vi "Associated Power Technologies 8500 Series List Mode.vi"() -> ()   [LabVIEW 2014]
doc: "This VI is an example for controlling the power source, APT-8500 series, of Associated Power Technologies. \n\nThe list mode which behave the configured sequences step by step is one of the operation mode on APT8500. This VI is an example showing how many configurations need to be set up."
uses:
  <instrlib>/Associated Power Technologies 8500 Series/Public/Configure/List Mode/List Mode - Delete File.vi
  <instrlib>/Associated Power Technologies 8500 Series/Public/Configure/List Mode/List Mode - Add File.vi
  <instrlib>/Associated Power Technologies 8500 Series/Public/Configure/List Mode/List Mode - Edit File.vi
  <instrlib>/Associated Power Technologies 8500 Series/Public/Configure/List Mode/List Mode - Configure File Loop.vi
  <instrlib>/Associated Power Technologies 8500 Series/Public/Configure/List Mode/List Mode - Configure Trigger Source.vi
  <instrlib>/Associated Power Technologies 8500 Series/Public/Configure/List Mode/List Mode - Configure Base.vi
  <instrlib>/Associated Power Technologies 8500 Series/Public/Configure/List Mode/List Mode - Configure Range.vi
  <instrlib>/Associated Power Technologies 8500 Series/Public/Configure/List Mode/List Mode - Configure General AC Voltage.vi
  <instrlib>/Associated Power Technologies 8500 Series/Public/Configure/List Mode/List Mode - Configure General Frequency.vi
  <instrlib>/Associated Power Technologies 8500 Series/Public/Configure/List Mode/List Mode - Configure General DC Voltage.vi
  <instrlib>/Associated Power Technologies 8500 Series/Public/Configure/List Mode/List Mode - Configure Phase Connection.vi
  <instrlib>/Associated Power Technologies 8500 Series/Public/Configure/List Mode/List Mode - Seq - Add Sequence.vi
  <instrlib>/Associated Power Technologies 8500 Series/Public/Configure/List Mode/List Mode - Seq - Edit Sequence.vi
  <instrlib>/Associated Power Technologies 8500 Series/Public/Configure/List Mode/List Mode - Seq - Configure Output Waveform.vi
  <instrlib>/Associated Power Technologies 8500 Series/Public/Configure/List Mode/List Mode - Seq - Configure Start Angle.vi
  <instrlib>/Associated Power Technologies 8500 Series/Public/Configure/List Mode/List Mode - Seq - Configure Start AC Voltage.vi
  <instrlib>/Associated Power Technologies 8500 Series/Public/Configure/List Mode/List Mode - Seq - Configure Start Frequency.vi
  <instrlib>/Associated Power Technologies 8500 Series/Public/Configure/List Mode/List Mode - Seq - Configure Start DC Voltage.vi
  <instrlib>/Associated Power Technologies 8500 Series/Public/Configure/List Mode/List Mode - Seq - Configure End AC Voltage.vi
  <instrlib>/Associated Power Technologies 8500 Series/Public/Configure/List Mode/List Mode - Seq - Configure End Frequency.vi
  <instrlib>/Associated Power Technologies 8500 Series/Public/Configure/List Mode/List Mode - Seq - Configure End DC Voltage.vi
  <instrlib>/Associated Power Technologies 8500 Series/Public/Configure/List Mode/List Mode - Seq - Configure Cycle.vi
  <instrlib>/Associated Power Technologies 8500 Series/Public/Configure/List Mode/List Mode - Seq - Configure Dwell Time.vi
  <instrlib>/Associated Power Technologies 8500 Series/Public/Configure/List Mode/List Mode - Seq - Configure Time Unit.vi
  <instrlib>/Associated Power Technologies 8500 Series/Public/Configure/List Mode/List Mode - Seq - Configure Limitation Delay Time.vi
  <instrlib>/Associated Power Technologies 8500 Series/Public/Configure/List Mode/List Mode - Seq - Configure THD.vi
  <instrlib>/Associated Power Technologies 8500 Series/Public/Configure/List Mode/List Mode - Seq - Configure Current High Limitation.vi
  <instrlib>/Associated Power Technologies 8500 Series/Public/Configure/List Mode/List Mode - Seq - Configure Current Low Limitation.vi
  <instrlib>/Associated Power Technologies 8500 Series/Public/Configure/List Mode/List Mode - Seq - Configure Power High Limitation.vi
  <instrlib>/Associated Power Technologies 8500 Series/Public/Configure/List Mode/List Mode - Seq - Configure Power Low Limitation.vi
  <instrlib>/Associated Power Technologies 8500 Series/Public/Configure/List Mode/List Mode - Seq - Configure PF High Limitation.vi
  <instrlib>/Associated Power Technologies 8500 Series/Public/Configure/List Mode/List Mode - Seq - Configure PF Low Limitation.vi
  <instrlib>/Associated Power Technologies 8500 Series/Public/Configure/List Mode/List Mode - Seq - Configure Current Peak High Limitation.vi
  <instrlib>/Associated Power Technologies 8500 Series/Public/Configure/List Mode/List Mode - Seq - Configure Current Peak Low Limitation.vi
  <instrlib>/Associated Power Technologies 8500 Series/Public/Configure/List Mode/List Mode - Seq - Configure Reactive Power High Limitation.vi
  <instrlib>/Associated Power Technologies 8500 Series/Public/Configure/List Mode/List Mode - Seq - Configure Reactive Power Low Limitation.vi
  <instrlib>/Associated Power Technologies 8500 Series/Public/Configure/List Mode/List Mode - Seq - Configure Crest Factor High Limitation.vi
  <instrlib>/Associated Power Technologies 8500 Series/Public/Configure/List Mode/List Mode - Seq - Configure Crest Factor Low Limitation.vi
  <instrlib>/Associated Power Technologies 8500 Series/Public/Configure/List Mode/List Mode - Seq - Configure Apparent Power High Limitation.vi
  <instrlib>/Associated Power Technologies 8500 Series/Public/Configure/List Mode/List Mode - Seq - Configure Apparent Power Low Limitation.vi
  <instrlib>/Associated Power Technologies 8500 Series/Associated Power Technologies 8500 Series.lvlib
panel:
  in  "Sequences Array":T1(array[cluster])=[{"Waveform Type"=0, "Start Angle(degree)"=90, "Start AC Voltage"=100.0, "Start Frequency"=50.0, "Start DC Voltage"=0.0, "End AC Voltage"=120.0, "End Frequency"=60.0, "End DC Voltage"=0.0, "Cycles"=9999, "Dwell Time"=1.0, "Unit"=1, "Delay Time"=1.0, "THD"=0.0, "Limits"={"A-HI"=0.0, "A-LO"=0.0, "P-HI"=0, "P-LO"=0, "PF-HI"=0.0, "PF-LO"=0.0, "Apk-HI"=0.0, "Apk-LO"=0.0, "Q-HI"=0, "Q-LO"=0, "CF-HI"=0.0, "CF-LO"=0.0, "VA-HI"=0.0, "VA-LO"=0.0}}] {"Waveform Type" items=["Sine", "Triangle", "Square", "Clipped"]; "Start Angle(degree)" max=359; "Start AC Voltage" min=0.0 max=310.0; "Start Frequency" min=5.0 max=1200.0; "Start DC Voltage" min=0.0 max=420.0; "End AC Voltage" min=0.0 max=310.0; "End Frequency" min=5.0 max=1200.0; "End DC Voltage" min=0.0 max=420.0; "Cycles" min=1 max=9999; "Dwell Time" min=1.0 max=999.9 step=0.1; "Unit" items=["MS", "SECOND", "MINUTE", "HOUR"]; "Delay Time" min=0.0 max=999.9 step=0.1; "THD" min=0.0 max=46.0 step=0.1}
  in  "Program Setup":T2={"Loop Count"=1, "Trigger Source"=0, "Base"=1, "Range"=0, "AC Voltage"=100.0, "Frequency"=60.0, "DC Voltage"=0.0, "Phase Connection"=0} {"Loop Count" max=50000; "Trigger Source" items=["AUTO", "MANUAL"]; "Base" items=["TIME", "CYCLE"]; "Range" items=["AUTO", "HIGH", "LOW"]; "AC Voltage" min=0.0 max=310.0; "Frequency" min=5.0 max=1200.0; "DC Voltage" min=0.0 max=420.0; "Phase Connection" items=["OFF", "ON"]}
  in  "File Name":string="EXAMPLE"
  in  "Serial Configuration":T3={"Baud Rate"=115200, "Parity"=0, "Data Bits"=8, "Stop Bits"=10, "Flow Control"=0} {"Flow Control" items=["None", "XON/XOFF", "RTS/CTS", "XON/XOFF & RTS/CTS", "DTR/DSR", "XON/XOFF & DTR/DSR"]; "Stop Bits" items=["1.0"=10, "1.5"=15, "2.0"=20]; "Data Bits" items=["7"=7, "8"=8]; "Parity" items=["None", "Odd", "Even", "Mark", "Space"]; "Baud Rate" items=["300"=300, "600"=600, "1200"=1200, "2400"=2400, "4800"=4800, "9600"=9600, "19200"=19200, "38400"=38400, "115200"=115200]}
  in  "VISA resource name":refnum<visa-resource-name>
  # "Create List Mode File of APT-8500 Series"
  # "This program is to explain how to build up a List Mode file and configure the parameters."
  # "Initialization"
  # "Configurations"
  # "(c) 2020 Associated Power Technologies.  ALL RIGHTS RESERVED."
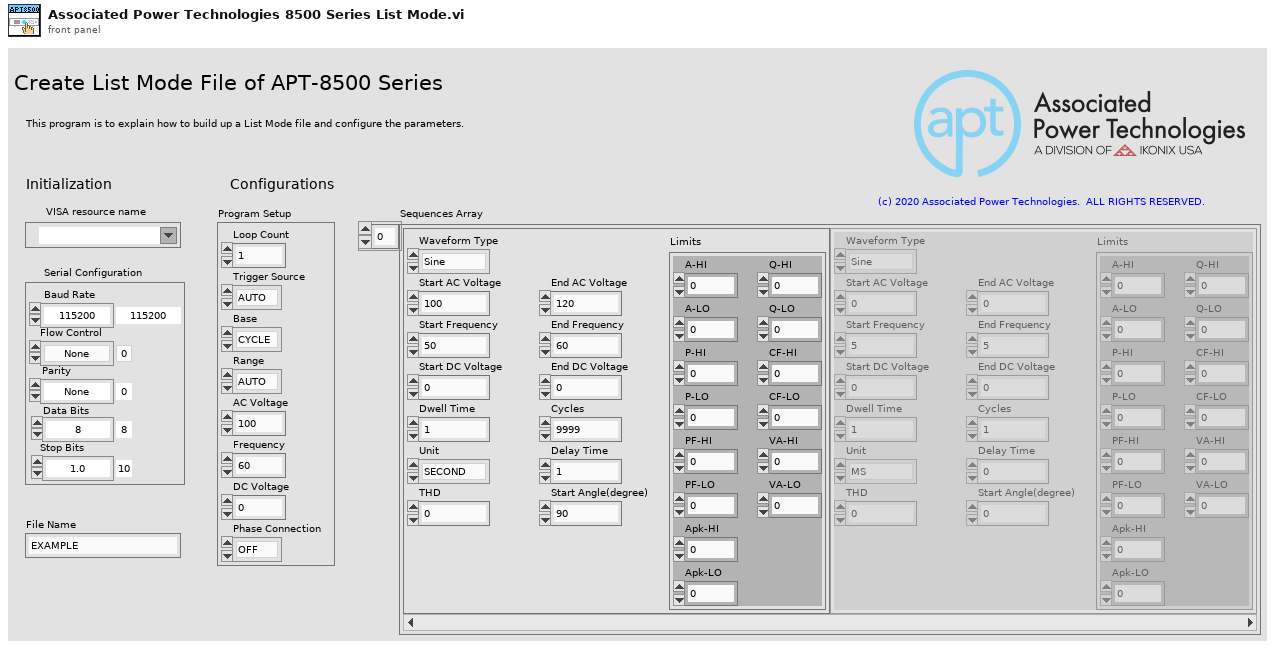
[diagram p1: front panel]
types:
  T1 = cluster{"Waveform Type":u16, "Start Angle(degree)":u16, "Start AC Voltage":dbl, "Start Frequency":dbl, "Start DC Voltage":dbl, "End AC Voltage":dbl, "End Frequency":dbl, "End DC Voltage":dbl, "Cycles":u32, "Dwell Time":dbl, "Unit":u16, "Delay Time":dbl, "THD":dbl, "Limits":cluster{"A-HI":dbl, "A-LO":dbl, "P-HI":u32, "P-LO":u32, "PF-HI":dbl, "PF-LO":dbl, "Apk-HI":dbl, "Apk-LO":dbl, "Q-HI":u32, "Q-LO":u32, "CF-HI":dbl, "CF-LO":dbl, "VA-HI":dbl, "VA-LO":dbl}}[]
  T2 = cluster{"Loop Count":u16, "Trigger Source":u16, "Base":u16, "Range":u16, "AC Voltage":dbl, "Frequency":dbl, "DC Voltage":dbl, "Phase Connection":u16}
  T3 = cluster{"Baud Rate":u32, "Parity":u16, "Data Bits":u16, "Stop Bits":u16, "Flow Control":u16}
  T4 = cluster{"A-HI":dbl, "A-LO":dbl, "P-HI":u32, "P-LO":u32, "PF-HI":dbl, "PF-LO":dbl, "Apk-HI":dbl, "Apk-LO":dbl, "Q-HI":u32, "Q-LO":u32, "CF-HI":dbl, "CF-LO":dbl, "VA-HI":dbl, "VA-LO":dbl}
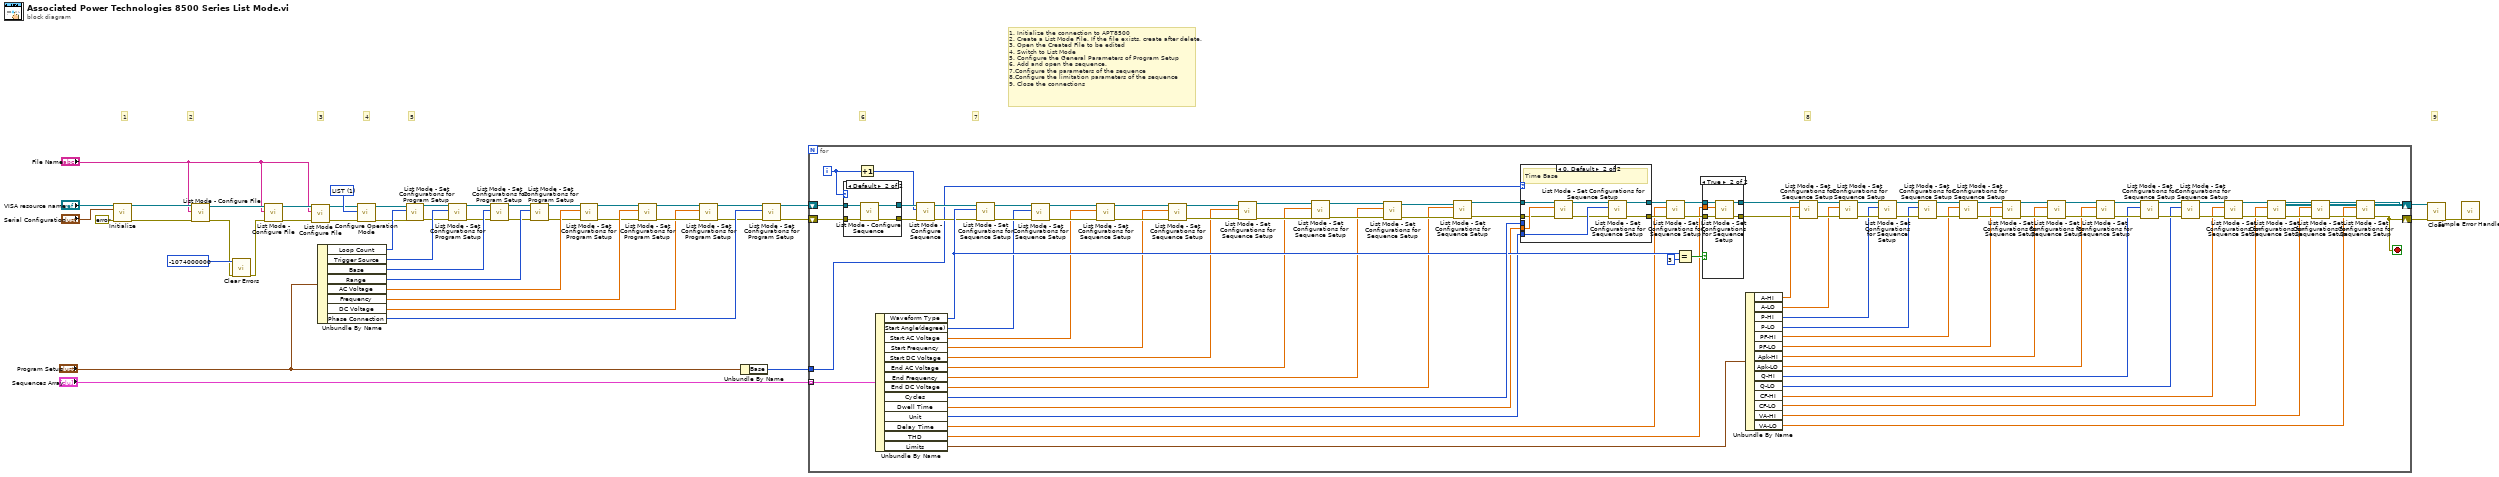
[diagram p0: block diagram]
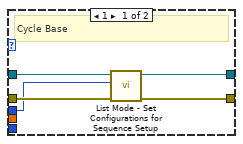
[diagram p2: hidden frame]
diagram:
  w32 = u16 1 items=["MANUAL", "LIST", "PULSE", "STEP"] ("Operation Mode")
  # "9"
  # "4"
  # "8"
  # "7"
  # "6"
  # "1. Initialize the connection to APT8500\n2. Create a List Mode File. If the file exists, create after delete. \n3. Open the Created File to be edited\n4. Switch to List Mode \n5. Configure the General Parameters of Program Setup\n6. Add and open the sequence.\n7.Configure the parameters of the sequence\n8.Configure the limitation parameters of the sequence\n9. Close the connections"
  # "5"
  # "3"
  # "2"
  # "1"
  n1 = call <instrlib>:"Initialize.vi"("VISA resource name"="VISA resource name", "Serial Configuration"="Serial Configuration", "error in (no error)"=errorcluster {"status"=FALSE, "code"=0, "source"=""}) -> ("VISA resource name out"=w40:refnum<visa-resource-name>, "error out"=w38:errorcluster)  [unwired: 11 in]
  n2 = call-poly <instrlib>:"List Mode - Configure File.vi"("error in (no error)"=w38, "File Name"="File Name", "VISA resource name"=w40) -> ("error out"=w36:errorcluster, "VISA resource name out"=w39:refnum<visa-resource-name>)  [unwired: 7 in]
  n3 = call <vilib>:"Clear Errors.vi"("error in (no error)"=w36, "specific error code to clear (0: all)"=-1074000000) -> ("error out"=w35:errorcluster)  [unwired: 4 in, 1 out]
  n4 = call-poly <instrlib>:"List Mode - Configure File.vi"("error in (no error)"=w35, "File Name"="File Name", "VISA resource name"=w39) -> ("error out"=w34:errorcluster, "VISA resource name out"=w43:refnum<visa-resource-name>)  [unwired: 7 in]
  n5 = call-poly <instrlib>:"List Mode - Configure File.vi"("error in (no error)"=w34, "File Name"="File Name", "VISA resource name"=w43) -> ("error out"=w30:errorcluster, "VISA resource name out"=w31:refnum<visa-resource-name>)  [unwired: 7 in]
  n6 = Unbundle By Name("Program Setup") -> ("Loop Count"=w21:u16, "Trigger Source"=w22:u16, "Base"=w23:u16, "Range"=w24:u16, "AC Voltage"=w25:dbl, "Frequency"=w26:dbl, "DC Voltage"=w6:dbl, "Phase Connection"=w27:u16)
  n7 = call <instrlib>:"Configure Operation Mode.vi"("error in (no error)"=w30, "Operation Mode (MANUAL)"=w32, "VISA resource name"=w31) -> ("error out"=w4:errorcluster, "VISA resource name out"=w5:refnum<visa-resource-name>)  [unwired: 7 in]
  n8 = call-poly <instrlib>:"List Mode - Set Configurations for Program Setup.vi"("error in (no error)"=w4, "Loop Count"=w21, "VISA resource name"=w5) -> ("error out"=w7:errorcluster, "VISA resource name out"=w14:refnum<visa-resource-name>)  [unwired: 7 in]
  n9 = call-poly <instrlib>:"List Mode - Set Configurations for Program Setup.vi"("error in (no error)"=w7, "Trigger Source"=w22, "VISA resource name"=w14) -> ("error out"=w8:errorcluster, "VISA resource name out"=w15:refnum<visa-resource-name>)  [unwired: 7 in]
  n10 = call-poly <instrlib>:"List Mode - Set Configurations for Program Setup.vi"("error in (no error)"=w8, "Base"=w23, "VISA resource name"=w15) -> ("error out"=w9:errorcluster, "VISA resource name out"=w16:refnum<visa-resource-name>)  [unwired: 7 in]
  n11 = call-poly <instrlib>:"List Mode - Set Configurations for Program Setup.vi"("error in (no error)"=w9, "Range"=w24, "VISA resource name"=w16) -> ("error out"=w10:errorcluster, "VISA resource name out"=w17:refnum<visa-resource-name>)  [unwired: 7 in]
  n12 = call-poly <instrlib>:"List Mode - Set Configurations for Program Setup.vi"("error in (no error)"=w10, "AC Voltage"=w25, "VISA resource name"=w17) -> ("error out"=w11:errorcluster, "VISA resource name out"=w18:refnum<visa-resource-name>)  [unwired: 7 in]
  n13 = call-poly <instrlib>:"List Mode - Set Configurations for Program Setup.vi"("error in (no error)"=w11, "Frequency (60)"=w26, "VISA resource name"=w18) -> ("error out"=w12:errorcluster, "VISA resource name out"=w19:refnum<visa-resource-name>)  [unwired: 7 in]
  n14 = call-poly <instrlib>:"List Mode - Set Configurations for Program Setup.vi"("error in (no error)"=w12, "DC Voltage"=w6, "VISA resource name"=w19) -> ("error out"=w13:errorcluster, "VISA resource name out"=w20:refnum<visa-resource-name>)  [unwired: 7 in]
  n15 = Unbundle By Name("Program Setup") -> ("Base"=w41:u16)
  n16 = call-poly <instrlib>:"List Mode - Set Configurations for Program Setup.vi"("error in (no error)"=w13, "Phase Connection"=w27, "VISA resource name"=w20) -> ("error out"=w1:errorcluster, "VISA resource name out"=w2:refnum<visa-resource-name>)  [unwired: 7 in]
  n17 = for {
    shift-right: [w48] -> w28
    shift-left: w2 -> [w137]
    shift-right: [w49] -> w29
    shift-left: w1 -> [w136]
    tunnel: "Sequences Array" -> [w94] mode=indexing
    tunnel: w41 -> [w93]
    i -> [w133]
    stop <- w49 stop-if-true
    n18 = case shown="Default" w133 {
      tunnel: w137 -> [w158 w163]
      tunnel: w136 -> [w159 w162]
      tunnel: [w158 w161] -> w135
      tunnel: [w159 w160] -> w134
      frame 0 {
      }
      frame Default {
        n19 = call-poly <instrlib>:"List Mode - Configure Sequence.vi"("error in (no error)"=w162, "VISA resource name"=w163) -> ("error out"=w160:errorcluster, "VISA resource name out"=w161:refnum<visa-resource-name>)  [unwired: 8 in]
      }
    }
    n20 = Increment(x=w133) -> (x+1=w132:i32)
    n21 = Unbundle By Name(w94) -> ("Waveform Type"=w126:u16, "Start Angle(degree)"=w123:u16, "Start AC Voltage"=w120:dbl, "Start Frequency"=w117:dbl, "Start DC Voltage"=w114:dbl, "End AC Voltage"=w107:dbl, "End Frequency"=w106:dbl, "End DC Voltage"=w105:dbl, "Cycles"=w131:u32, "Dwell Time"=w104:dbl, "Unit"=w103:u16, "Delay Time"=w98:dbl, "THD"=w97:dbl, "Limits"=w50:T4)
    n22 = call-poly <instrlib>:"List Mode - Configure Sequence.vi"("error in (no error)"=w134, "Sequence index"=w132, "VISA resource name"=w135) -> ("error out"=w95:errorcluster, "VISA resource name out"=w96:refnum<visa-resource-name>)  [unwired: 7 in]
    n23 = call-poly <instrlib>:"List Mode - Set Configurations for Sequence Setup.vi"("error in (no error)"=w95, "Waveform Type"=w126, "VISA resource name"=w96) -> ("error out"=w124:errorcluster, "VISA resource name out"=w125:refnum<visa-resource-name>)  [unwired: 7 in]
    n24 = call-poly <instrlib>:"List Mode - Set Configurations for Sequence Setup.vi"("error in (no error)"=w124, "Start Angle(degree)"=w123, "VISA resource name"=w125) -> ("error out"=w121:errorcluster, "VISA resource name out"=w122:refnum<visa-resource-name>)  [unwired: 7 in]
    n25 = call-poly <instrlib>:"List Mode - Set Configurations for Sequence Setup.vi"("error in (no error)"=w121, "Start AC Voltage"=w120, "VISA resource name"=w122) -> ("error out"=w118:errorcluster, "VISA resource name out"=w119:refnum<visa-resource-name>)  [unwired: 7 in]
    n26 = call-poly <instrlib>:"List Mode - Set Configurations for Sequence Setup.vi"("error in (no error)"=w118, "Start Frequency"=w117, "VISA resource name"=w119) -> ("error out"=w115:errorcluster, "VISA resource name out"=w116:refnum<visa-resource-name>)  [unwired: 7 in]
    n27 = call-poly <instrlib>:"List Mode - Set Configurations for Sequence Setup.vi"("error in (no error)"=w115, "Start DC Voltage"=w114, "VISA resource name"=w116) -> ("error out"=w110:errorcluster, "VISA resource name out"=w113:refnum<visa-resource-name>)  [unwired: 7 in]
    n28 = call-poly <instrlib>:"List Mode - Set Configurations for Sequence Setup.vi"("error in (no error)"=w110, "End AC Voltage"=w107, "VISA resource name"=w113) -> ("error out"=w109:errorcluster, "VISA resource name out"=w112:refnum<visa-resource-name>)  [unwired: 7 in]
    n29 = call-poly <instrlib>:"List Mode - Set Configurations for Sequence Setup.vi"("error in (no error)"=w109, "End Frequency"=w106, "VISA resource name"=w112) -> ("error out"=w108:errorcluster, "VISA resource name out"=w111:refnum<visa-resource-name>)  [unwired: 7 in]
    n30 = call-poly <instrlib>:"List Mode - Set Configurations for Sequence Setup.vi"("error in (no error)"=w108, "End DC Voltage"=w105, "VISA resource name"=w111) -> ("error out"=w130:errorcluster, "VISA resource name out"=w129:refnum<visa-resource-name>)  [unwired: 7 in]
    n31 = case shown="0, Default" w93 {
      tunnel: [w139 w150] -> w101
      tunnel: [w140 w149] -> w102
      tunnel: w103 -> [_ w148]
      tunnel: w104 -> [_ w147]
      tunnel: w130 -> [w141 w145]
      tunnel: w129 -> [w142 w143]
      tunnel: w131 -> [w138 _]
      frame 1 {
        # "Cycle Base"
        n32 = call-poly <instrlib>:"List Mode - Set Configurations for Sequence Setup.vi"("error in (no error)"=w141, "Cycles"=w138, "VISA resource name"=w142) -> ("error out"=w139:errorcluster, "VISA resource name out"=w140:refnum<visa-resource-name>)  [unwired: 7 in]
      }
      frame 0, Default {
        # "Time Base"
        n33 = call-poly <instrlib>:"List Mode - Set Configurations for Sequence Setup.vi"("error in (no error)"=w145, "Dwell Time"=w147, "VISA resource name"=w143) -> ("error out"=w146:errorcluster, "VISA resource name out"=w144:refnum<visa-resource-name>)  [unwired: 7 in]
        n34 = call-poly <instrlib>:"List Mode - Set Configurations for Sequence Setup.vi"("error in (no error)"=w146, "Unit"=w148, "VISA resource name"=w144) -> ("error out"=w150:errorcluster, "VISA resource name out"=w149:refnum<visa-resource-name>)  [unwired: 7 in]
      }
    }
    n35 = call-poly <instrlib>:"List Mode - Set Configurations for Sequence Setup.vi"("error in (no error)"=w101, "Delay Time"=w98, "VISA resource name"=w102) -> ("error out"=w99:errorcluster, "VISA resource name out"=w100:refnum<visa-resource-name>)  [unwired: 7 in]
    n36 = Equal?(x=w126, y=u16 3) -> (x = y?=w128:bool)
    n37 = case shown="True" w128 {
      tunnel: [w151 w157] -> w51
      tunnel: [w152 w156] -> w52
      tunnel: w97 -> [_ w155]
      tunnel: w99 -> [w151 w154]
      tunnel: w100 -> [w152 w153]
      frame False {
      }
      frame True {
        n38 = call-poly <instrlib>:"List Mode - Set Configurations for Sequence Setup.vi"("error in (no error)"=w154, "THD"=w155, "VISA resource name"=w153) -> ("error out"=w157:errorcluster, "VISA resource name out"=w156:refnum<visa-resource-name>)  [unwired: 7 in]
      }
    }
    n39 = Unbundle By Name(w50) -> ("A-HI"=w66:dbl, "A-LO"=w65:dbl, "P-HI"=w64:u32, "P-LO"=w63:u32, "PF-HI"=w62:dbl, "PF-LO"=w61:dbl, "Apk-HI"=w60:dbl, "Apk-LO"=w59:dbl, "Q-HI"=w58:u32, "Q-LO"=w57:u32, "CF-HI"=w56:dbl, "CF-LO"=w55:dbl, "VA-HI"=w54:dbl, "VA-LO"=w53:dbl)
    n40 = call-poly <instrlib>:"List Mode - Set Configurations for Sequence Setup.vi"("error in (no error)"=w51, "A-HI"=w66, "VISA resource name"=w52) -> ("error out"=w67:errorcluster, "VISA resource name out"=w92:refnum<visa-resource-name>)  [unwired: 7 in]
    n41 = call-poly <instrlib>:"List Mode - Set Configurations for Sequence Setup.vi"("error in (no error)"=w67, "A-LO"=w65, "VISA resource name"=w92) -> ("error out"=w68:errorcluster, "VISA resource name out"=w91:refnum<visa-resource-name>)  [unwired: 7 in]
    n42 = call-poly <instrlib>:"List Mode - Set Configurations for Sequence Setup.vi"("error in (no error)"=w68, "P-HI"=w64, "VISA resource name"=w91) -> ("error out"=w69:errorcluster, "VISA resource name out"=w90:refnum<visa-resource-name>)  [unwired: 7 in]
    n43 = call-poly <instrlib>:"List Mode - Set Configurations for Sequence Setup.vi"("error in (no error)"=w69, "P-LO"=w63, "VISA resource name"=w90) -> ("error out"=w70:errorcluster, "VISA resource name out"=w89:refnum<visa-resource-name>)  [unwired: 7 in]
    n44 = call-poly <instrlib>:"List Mode - Set Configurations for Sequence Setup.vi"("error in (no error)"=w70, "PF-HI"=w62, "VISA resource name"=w89) -> ("error out"=w71:errorcluster, "VISA resource name out"=w88:refnum<visa-resource-name>)  [unwired: 7 in]
    n45 = call-poly <instrlib>:"List Mode - Set Configurations for Sequence Setup.vi"("error in (no error)"=w71, "PF-LO"=w61, "VISA resource name"=w88) -> ("error out"=w72:errorcluster, "VISA resource name out"=w87:refnum<visa-resource-name>)  [unwired: 7 in]
    n46 = call-poly <instrlib>:"List Mode - Set Configurations for Sequence Setup.vi"("error in (no error)"=w72, "Apk-HI"=w60, "VISA resource name"=w87) -> ("error out"=w73:errorcluster, "VISA resource name out"=w86:refnum<visa-resource-name>)  [unwired: 7 in]
    n47 = call-poly <instrlib>:"List Mode - Set Configurations for Sequence Setup.vi"("error in (no error)"=w73, "Apk-LO"=w59, "VISA resource name"=w86) -> ("error out"=w74:errorcluster, "VISA resource name out"=w85:refnum<visa-resource-name>)  [unwired: 7 in]
    n48 = call-poly <instrlib>:"List Mode - Set Configurations for Sequence Setup.vi"("error in (no error)"=w74, "Q-HI"=w58, "VISA resource name"=w85) -> ("error out"=w75:errorcluster, "VISA resource name out"=w84:refnum<visa-resource-name>)  [unwired: 7 in]
    n49 = call-poly <instrlib>:"List Mode - Set Configurations for Sequence Setup.vi"("error in (no error)"=w75, "Q-LO"=w57, "VISA resource name"=w84) -> ("error out"=w76:errorcluster, "VISA resource name out"=w83:refnum<visa-resource-name>)  [unwired: 7 in]
    n50 = call-poly <instrlib>:"List Mode - Set Configurations for Sequence Setup.vi"("error in (no error)"=w76, "CF-HI"=w56, "VISA resource name"=w83) -> ("error out"=w77:errorcluster, "VISA resource name out"=w82:refnum<visa-resource-name>)  [unwired: 7 in]
    n51 = call-poly <instrlib>:"List Mode - Set Configurations for Sequence Setup.vi"("error in (no error)"=w77, "CF-LO"=w55, "VISA resource name"=w82) -> ("error out"=w78:errorcluster, "VISA resource name out"=w81:refnum<visa-resource-name>)  [unwired: 7 in]
    n52 = call-poly <instrlib>:"List Mode - Set Configurations for Sequence Setup.vi"("error in (no error)"=w78, "VA-HI"=w54, "VISA resource name"=w81) -> ("error out"=w79:errorcluster, "VISA resource name out"=w80:refnum<visa-resource-name>)  [unwired: 7 in]
    n53 = call-poly <instrlib>:"List Mode - Set Configurations for Sequence Setup.vi"("error in (no error)"=w79, "VA-LO"=w53, "VISA resource name"=w80) -> ("error out"=w49:errorcluster, "VISA resource name out"=w48:refnum<visa-resource-name>)  [unwired: 7 in]
  }
  n54 = call <instrlib>:"Close.vi"("VISA resource name"=w28, "error in (no error)"=w29) -> ("error out"=w33:errorcluster)  [unwired: 13 in]
  n55 = call <vilib>:"Simple Error Handler.vi"("error in (no error)"=w33) -> ()  [unwired: 4 in, 5 out]
